vi "Check four front leds.vi"(6 "VISA resource name":refnum<visa-resource-name>="COM5", 7 "Passed so far":bool, 8 "error in (no error)":errorcluster) -> (0 "error out":errorcluster, 4 "VISA Refnum out":refnum<visa-resource-name>, 5 "Passed?":bool)   [LabVIEW 2024]
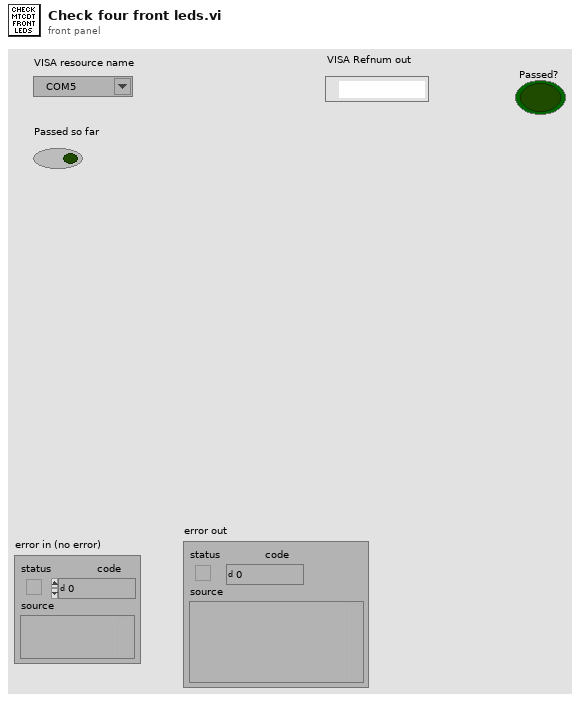
[diagram p1: front panel]
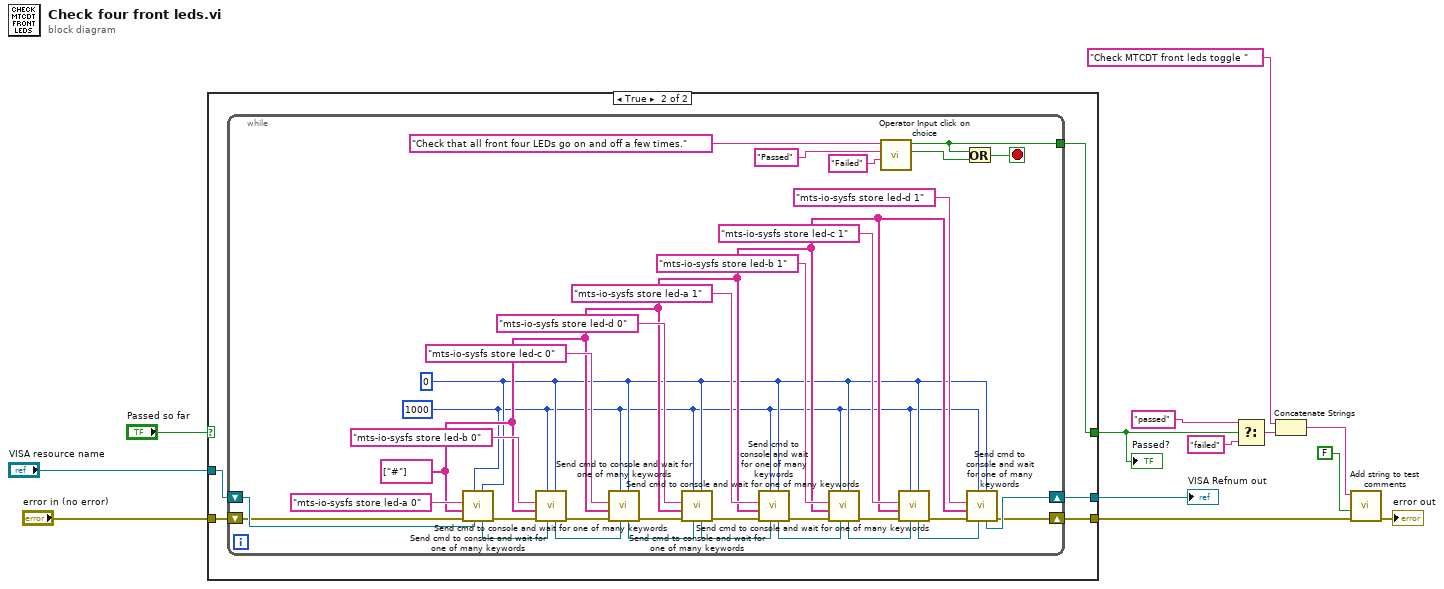
[diagram p0: block diagram]
diagram:
  n1 = case shown="True" "Passed so far" {
    selector: "Passed so far" -> [w16 _]
    tunnel: "error in (no error)" -> [w15 w21]
    tunnel: [w15 w17] -> w2
    tunnel: "VISA resource name" -> [w14 w20]
    tunnel: [w16 w18] -> w5
    tunnel: [w14 w19] -> w3
    frame False {
    }
    frame True {
      n2 = while {
        shift-right: [w34] -> w19
        shift-left: w20 -> [w55]
        shift-right: [w22] -> w17
        shift-left: w21 -> [w29]
        tunnel: [w25] -> w18
        stop <- w23 stop-if-true
        w31 = u32 0 ("Wait msecs after cmd ends (500ms)")
        w33 = string[] ["#"] ("Wait for keywords")
        w30 = u32 1000 ("Timeout (mSecs)")
        n3 = call "Send cmd to console and wait for one of many keywords.vi"("Wait msecs after cmd ends (500ms)"=w31, "VISA resource name"=w55, "Timeout (1000 mSecs)"=w30, "error in (no error)"=w29, "Wait for keywords"=w33, "cmd"="mts-io-sysfs store led-a 0") -> ("error out"=w53:errorcluster, "VISA Refnum out"=w48:refnum<visa-resource-name>)  [unwired: 1 in, 3 out]
        n4 = call "Send cmd to console and wait for one of many keywords.vi"("Wait msecs after cmd ends (500ms)"=w31, "VISA resource name"=w48, "Timeout (1000 mSecs)"=w30, "error in (no error)"=w53, "Wait for keywords"=w33, "cmd"="mts-io-sysfs store led-b 0") -> ("error out"=w50:errorcluster, "VISA Refnum out"=w47:refnum<visa-resource-name>)  [unwired: 1 in, 3 out]
        n5 = call "Send cmd to console and wait for one of many keywords.vi"("Wait msecs after cmd ends (500ms)"=w31, "VISA resource name"=w47, "Timeout (1000 mSecs)"=w30, "error in (no error)"=w50, "Wait for keywords"=w33, "cmd"="mts-io-sysfs store led-c 0") -> ("error out"=w49:errorcluster, "VISA Refnum out"=w46:refnum<visa-resource-name>)  [unwired: 1 in, 3 out]
        n6 = call "Send cmd to console and wait for one of many keywords.vi"("Wait msecs after cmd ends (500ms)"=w31, "VISA resource name"=w46, "Timeout (1000 mSecs)"=w30, "error in (no error)"=w49, "Wait for keywords"=w33, "cmd"="mts-io-sysfs store led-d 0") -> ("error out"=w35:errorcluster, "VISA Refnum out"=w32:refnum<visa-resource-name>)  [unwired: 1 in, 3 out]
        n7 = call "Send cmd to console and wait for one of many keywords.vi"("Wait msecs after cmd ends (500ms)"=w31, "VISA resource name"=w32, "Timeout (1000 mSecs)"=w30, "error in (no error)"=w35, "Wait for keywords"=w33, "cmd"="mts-io-sysfs store led-a 1") -> ("error out"=w38:errorcluster, "VISA Refnum out"=w43:refnum<visa-resource-name>)  [unwired: 1 in, 3 out]
        n8 = call "Send cmd to console and wait for one of many keywords.vi"("Wait msecs after cmd ends (500ms)"=w31, "VISA resource name"=w43, "Timeout (1000 mSecs)"=w30, "error in (no error)"=w38, "Wait for keywords"=w33, "cmd"="mts-io-sysfs store led-b 1") -> ("error out"=w41:errorcluster, "VISA Refnum out"=w44:refnum<visa-resource-name>)  [unwired: 1 in, 3 out]
        n9 = call "Operator Input click on choice.vi"("button2 text"="Failed", "button1 text"="Passed", "Operator text"="Check that all front four LEDs go on and off a few times.") -> ("button2 clicked?"=w24:bool, "button1 clicked?"=w25:bool)  [unwired: 6 in, 1 out]
        n10 = call "Send cmd to console and wait for one of many keywords.vi"("Wait msecs after cmd ends (500ms)"=w31, "VISA resource name"=w44, "Timeout (1000 mSecs)"=w30, "error in (no error)"=w41, "Wait for keywords"=w33, "cmd"="mts-io-sysfs store led-c 1") -> ("error out"=w42:errorcluster, "VISA Refnum out"=w45:refnum<visa-resource-name>)  [unwired: 1 in, 3 out]
        n11 = Or(x=w25, y=w24) -> (x .or. y?=w23:bool)
        n12 = call "Send cmd to console and wait for one of many keywords.vi"("Wait msecs after cmd ends (500ms)"=w31, "VISA resource name"=w45, "Timeout (1000 mSecs)"=w30, "error in (no error)"=w42, "Wait for keywords"=w33, "cmd"="mts-io-sysfs store led-d 1") -> ("error out"=w22:errorcluster, "VISA Refnum out"=w34:refnum<visa-resource-name>)  [unwired: 1 in, 3 out]
      }
    }
  }
  "Passed?" <- w5
  "VISA Refnum out" <- w3
  n13 = Select(t="passed", s=w5, f="failed") -> (s? t:f=w9:string)
  n14 = Concatenate Strings("Check MTCDT front leds toggle " ("string"), w9) -> (w8:string)
  n15 = call "Add string to test comments.vi"("error in (no error)"=w2, "New Section (y)?"=FALSE, "Comments"=w8) -> ("error out"=→"error out":errorcluster)  [unwired: 7 in, 1 out]
